vi "Agilent 2000 3000 X-Series Adjacent Channel Power Ratio.vi"() -> ()   [LabVIEW 2015]
doc: "This example shows how to install an FFT analysis Adjacent Channel Power Ratio (ACPR) measurement on screen. \n\nNote:\nThis VI is not applicable for DSOX/MSOX 3000G Series model"
uses:
  Agilent 2000 3000 X-Series.lvlib
  Public/Configure/Math/Configure Math Function (FFT).vi
  Public/Configure/FFT/Configure FFT Measurement (Adjacent Channel Power Ratio).vi
panel:
  in  "Measurement Source (0: Function 1)":i32(ring) items=["Function 1", "Function 2", "Function 3", "Function 4", "Math 1", "Math 2", "Math 3", "Math 4", "FFT"]
  in  "Sideband (0: Center)":i32(ring) items=["Center", "High 1", "High 2", "High 3", "High 4", "High 5", "Low 1", "Low 2", "Low 3", "Low 4", "Low 5"]
  in  "Channel Spacing (50000 Hz)":dbl=50000.0
  in  "Channel Width (100000 Hz)":dbl=100000.0
  in  "Frequency Span (100000.0 Hz)":dbl=100000.0
  in  "Center Frequency (50000.0 Hz)":dbl=50000.0
  in  "Enable Display (T: Enable)":bool=TRUE
  in  "Math Operation (5: FFT)":i32(ring)=5 items=["Add", "Subtract", "Multiply", "Integrate", "Diff", "FFT", "SQRT", "Magnify", "Absolute", "Square", "LN", "LOG", "EXP", "TEN", "Lowpass", "Highpass", "Divide", "Linear", "Trend", "Btiming", "Bstate", "Envelope", "Smoothing", "Max Hold", "Min Hold", "Average", "Clock Recovery", "Peak", "FFT Phase", "MAX", "MIN"]
  in  "Math Function Index (1: Math Function 1)":i32(ring)=1 items=["Math Function 1"=1, "Math Function 2"=2, "Math Function 3"=3, "Math Function 4"=4]
  in  "Signal Source 1 (0: Channel 1)":i32(ring) items=["Channel 1", "Channel 2", "Channel 3", "Channel 4", "GOFT", "Bus 1", "Bus 2", "Function 1", "Function 2", "Function 3", "Math 1", "Math 2", "Math 3", "Waveform Memory 1", "Waveform Memory 2"]
  in  "VISA resource name":refnum<visa-resource-name>
  # "(c) 2018 - 2023 National Instruments.  ALL RIGHTS RESERVED."
  # "FFT Source Settings"
  # "FFT Measurement"
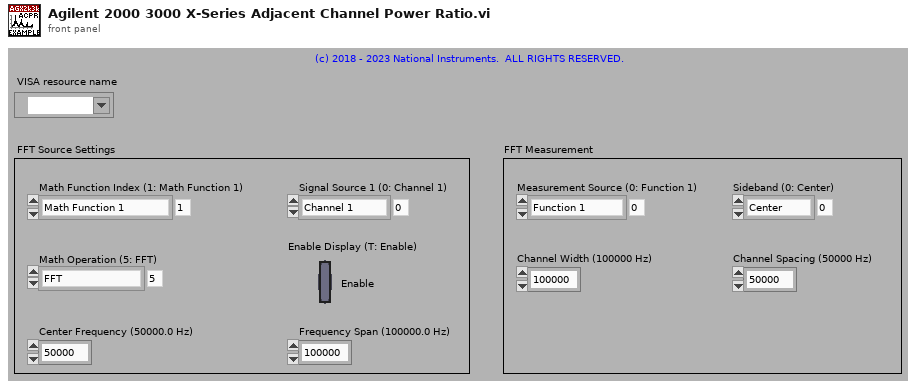
[diagram p1: front panel]
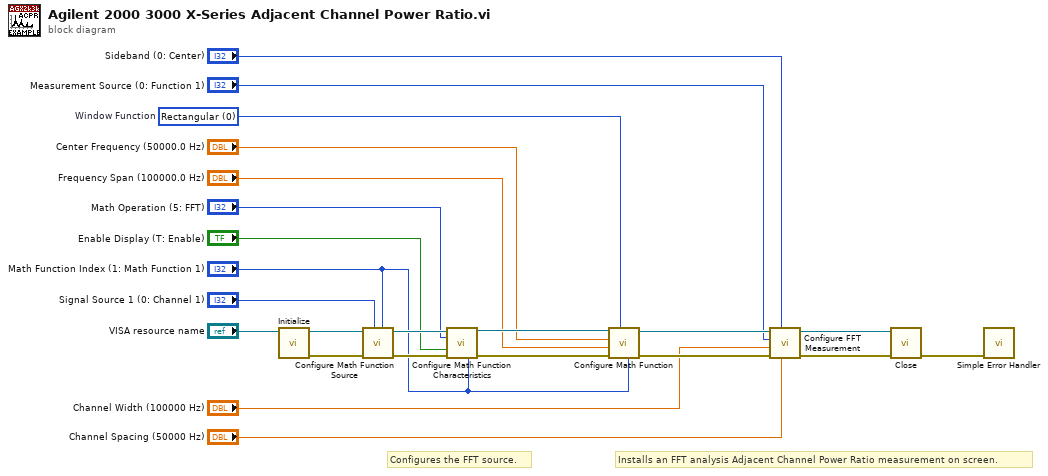
[diagram p0: block diagram]
diagram:
  w8 = 0 items=["Rectangular", "Hanning", "Flat Top", "Blackman-Harris"]  # Window Function
  # "Installs an FFT analysis Adjacent Channel Power Ratio measurement on screen."
  # "Configures the FFT source."
  n1 = call "Initialize.vi"("VISA resource name"="VISA resource name") -> ("error out"=w18:errorcluster, "VISA resource name out"=w23:refnum<visa-resource-name>)  [unwired: 9 in]
  n2 = call "Configure Math Function Source.vi"("Math Function Index (1: Math Function 1)"="Math Function Index (1: Math Function 1)", "Signal Source 1 (0: Channel 1)"="Signal Source 1 (0: Channel 1)", "error in (no error)"=w18, "VISA resource name"=w23) -> ("error out"=w17:errorcluster, "VISA resource name out"=w21:refnum<visa-resource-name>)  [unwired: 6 in]
  n3 = call "Configure Math Function Characteristics.vi"("VISA resource name"=w21, "Math Operation (0: Add)"="Math Operation (5: FFT)", "Enable Display (T: Enable)"="Enable Display (T: Enable)", "error in (no error)"=w17, "Math Function Index (1: Math Function 1)"="Math Function Index (1: Math Function 1)") -> ("VISA resource name out"=w20:refnum<visa-resource-name>, "error out"=w16:errorcluster)  [unwired: 9 in]
  n4 = call-poly "Configure Math Function.vi"("Math Function Index (1: Math Function 1)"="Math Function Index (1: Math Function 1)", "Window Function (0: Rectangular)"=w8, "error in (no error)"=w16, "Frequency Span (100000.0 Hz)"="Frequency Span (100000.0 Hz)", "Center Frequency (50000.0 Hz)"="Center Frequency (50000.0 Hz)", "VISA resource name"=w20) -> ("error out"=w15:errorcluster, "VISA resource name out"=w19:refnum<visa-resource-name>)  [unwired: 4 in]
  n5 = call-poly "Configure FFT Measurement.vi"("Channel Spacing (50000 Hz)"="Channel Spacing (50000 Hz)", "Sideband (0: Center)"="Sideband (0: Center)", "error in (no error)"=w15, "Channel Width (100000 Hz)"="Channel Width (100000 Hz)", "Measurement Source (0: Function 1)"="Measurement Source (0: Function 1)", "VISA resource name"=w19) -> ("error out"=w2:errorcluster, "VISA resource name out"=w3:refnum<visa-resource-name>)  [unwired: 4 in]
  n6 = call "Close.vi"("error in (no error)"=w2, "VISA resource name"=w3) -> ("error out"=w1:errorcluster)  [unwired: 9 in]
  n7 = call <vilib>:"Simple Error Handler.vi"("error in (no error)"=w1) -> ()  [unwired: 4 in, 5 out]
